vi "Set External Reference Clock.vi"(7 "Reference Frequency (10 MHz)":dbl=10000000.0 format="%#_13p", 8 "error in (no error)":errorcluster, 11 "reference":refnum<k15>) -> (0 "error out":errorcluster, 2 "PLL Lock Status":bool, 3 "reference out":refnum<k15>, 4 "Reference Clock Rate":dbl, 5 "Reference Clock Source":string)   [LabVIEW 2020, in "varilib.lvlib"]
doc: "Sets the clock source and clock rate for NI Scope Digitizer and reads them to verify correct setting."
uses:
  varilib.lvlib
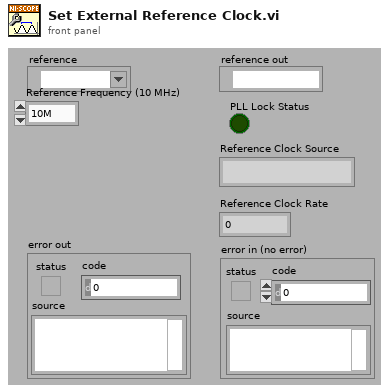
[diagram p1: front panel]
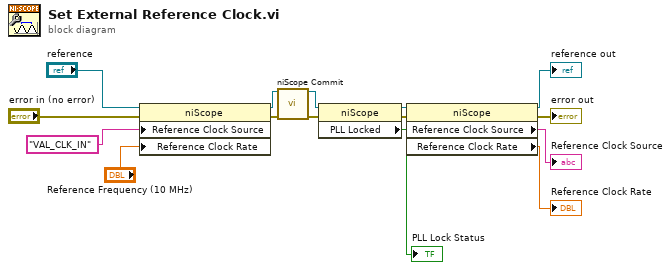
[diagram p0: block diagram]
diagram:
  n1 = property class="niScope"(reference="reference", error in="error in (no error)", "Reference Clock Source"="VAL_CLK_IN" ("Clocking:Reference (Input) Clock Source"), "Reference Clock Rate"="Reference Frequency (10 MHz)") -> (reference out=w7:refnum<k15>, error out=w6:errorcluster)
  n2 = call <instrlib>:"niScope Commit.vi"("instrument handle"=w7, "error in"=w6) -> ("instrument handle out"=w5:refnum<k15>, "error out"=w4:errorcluster)  [unwired: 12 in]
  n3 = property class="niScope"(reference=w5, error in=w4) -> (reference out=w12:refnum<k15>, error out=w11:errorcluster, "PLL Locked"=→"PLL Lock Status":bool)
  n4 = property class="niScope"(reference=w12, error in=w11) -> (reference out=→"reference out":refnum<k15>, error out=→"error out":errorcluster, "Reference Clock Source"=→"Reference Clock Source":string, "Reference Clock Rate"=→"Reference Clock Rate":dbl)
